vi "Pre Launch Init.vi"(11 "Graph in":refnum<class "Graph.lvclass">) -> (0 "error out":errorcluster, 3 "Graph out":refnum<class "Graph.lvclass">)   [LabVIEW 2020, in "Graph.lvlib" / "Graph.lvclass"]
doc: "(<B>Filename</B>: Actor Framework.lvlib:Actor.lvclass:Pre Launch Init.vi)\n\nDefines behavior that occurs after the Launch Nested Actor method is invoked but before the actor's Actor Core method begins running.\n\nThis implementation setups the data subscription and creates the user event for transfer of data to the UI."
uses:
  Graph.lvclass
  PPL/HDH.Actor Framework.Core.Actor.lvlibp/1abvi3w/vi.lib/ActorFramework/Message Enqueuer/Message Priority.ctl
  PPL/HDH.Data.Generic.lvlibp/Data.lvclass
  Graph.lvclass/Graph.ctl
  PPL/HDH.Actor Framework.Core.Actor.lvlibp/1abvi3w/vi.lib/ActorFramework/Actor/Actor.lvclass
  PPL/HDH.Actor Framework.Core.Publisher.lvlibp/Publisher Messages/Subscribe Msg/Subscribe Msg.lvclass
  PPL/HDH.Actor Framework.Core.Actor.lvlibp/1abvi3w/vi.lib/ActorFramework/Message Enqueuer/Message Enqueuer.lvclass
  C:/Current projects/WS/PPL/HDH.Actor Framework.Core.Actor.lvlibp/1abvi3w/vi.lib/ActorFramework/Actor/Actor.lvclass
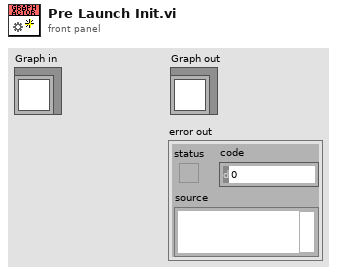
[diagram p1: front panel]
types:
  T1 = typedef "HDH.Actor Framework.Core.Actor.lvlibp/Message Enqueuer.lvclass/Message Priority.ctl" = enum16{"Low", "Normal", "High"}
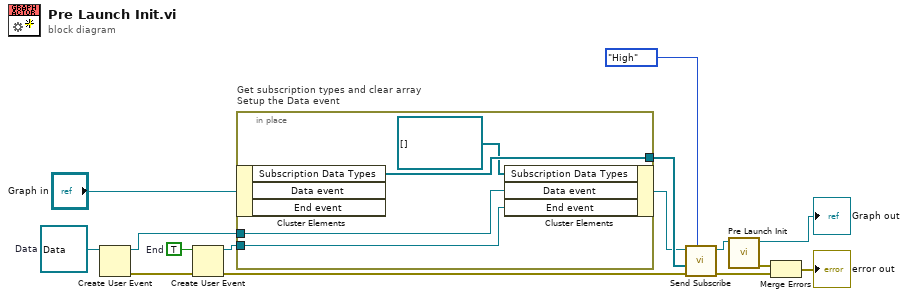
[diagram p0: block diagram]
diagram:
  w4 = TRUE  # End
  w6 = refnum<class "Data.lvclass"> refnum  # Data
  n1 = Create User Event(user event datatype=w6) -> (user event=w5:refnum<user-event>, error out=w3:errorcluster)  [unwired: 1 in]
  n2 = Create User Event(user event datatype=w4, error in=w3) -> (user event=w2:refnum<user-event>, error out=w1:errorcluster)
  n3 = in-place "Get subscription types and clear array\nSetup the Data event" {
    in-place-border: [w19] -> w10
    in-place-border: w5 -> [w17]
    in-place-border: w2 -> [w16]
    n4 = in-place-cluster #1("Graph in") -> ("Subscription Data Types"=w19:refnum<class "Data.lvclass">[])  [unwired: 2 out]
    n5 = in-place-cluster #1("Subscription Data Types"=refnum<class "Data.lvclass">[] [], "Data event"=w17, "End event"=w16) -> (w9:refnum<class "Graph.lvclass">)
  }
  n6 = call "Send Subscribe.vi"("Message Priority (High)"=Message_Priority."High", "error in (no error)"=w1, "Data Array"=w10, "Actor in"=w9) -> ("error out"=w7:errorcluster, "Actor out"=w12:refnum<class "Graph.lvclass">)  [unwired: 6 in]
  n7 = call-parent "Pre Launch Init.vi"("Actor in"=w12) -> ("error out"=w15:errorcluster, "Actor out"=→"Graph out":refnum<class "Graph.lvclass">)  [unwired: 9 in]
  n8 = Merge Errors(w15, w7) -> (→"error out":errorcluster)
